vi "libssh2_knownhost_init - invalid session - returns invalid known hosts collection.vi"() -> ()   [LabVIEW 2013, in "libssh2_tests.lvlib"]
uses:
  libssh2_tests.lvlib
  libssh2/Session Refnum.ctl
  libssh2/libssh2_init_default.vi
  <vilib>/addons/_JKI Toolkits/Caraya/classes/Assert/Assert True.vi
  libssh2/libssh2.lvlib
  <vilib>/addons/_JKI Toolkits/Caraya/classes/Test/Test.lvclass
  <vilib>/addons/_JKI Toolkits/Caraya/classes/Assert/Assert.lvclass
panel:
  out "error out":errorcluster
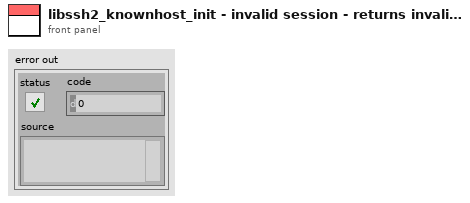
[diagram p1: front panel]
types:
  T1 = typedef "libssh2.lvlib/Session Refnum.ctl" = refnum<k1>
  T2 = typedef "libssh2.lvlib/Known Hosts Collection Refnum.ctl" = refnum<k1>
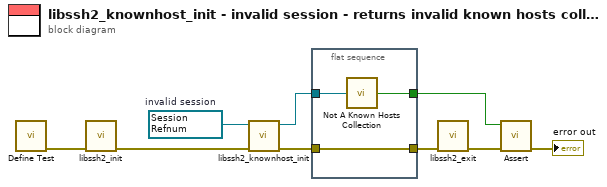
[diagram p0: block diagram]
diagram:
  w5 = T1 refnum items=["Session"]  # invalid session
  n1 = call <vilib>:"Define Test.vi"() -> ("error out"=w7:errorcluster)  [unwired: 10 in, 1 out]
  n2 = call-poly "libssh2_init.vi"("error in (no error)"=w7) -> ("error out"=w8:errorcluster)  [unwired: 10 in]
  n3 = call "libssh2_knownhost_init.vi"("error in (no error)"=w8, "session"=w5) -> ("error out"=w1:errorcluster, "known hosts collection"=w4:T2)  [unwired: 8 in]
  n4 = flat-sequence {
    tunnel: w4 -> [w12]
    tunnel: [w11] -> w3
    tunnel: [w10] -> w2
    tunnel: w1 -> [w10]
    frame #0 {
      n5 = call "Not A Known Hosts Collection.vi"("known hosts collection"=w12) -> ("Not a Known Hosts Collection?"=w11:bool)
    }
  }
  n6 = call "libssh2_exit.vi"("error in (no error)"=w2) -> ("error out"=w6:errorcluster)  [unwired: 10 in]
  n7 = call-poly <vilib>:"Assert.vi"("error in (no error)"=w6, "True?"=w3) -> ("error out"=→"error out":errorcluster)  [unwired: 8 in, 1 out]
